vi "overheat.vi"(8 "input valid":bool=TRUE, 9 "ready for output (T)":bool=TRUE, 10 "x":fxp<+/-,32,16>) -> (0 "output valid":bool, 1 "ready for input":bool, 2 "Output":fxp<+/-,32,16>)   [LabVIEW 2018]
uses:
  <vilib>/rvi/FXPMathLib/FxpDiv/subVIs/nifxpmath_Div_SimConfig.ctl
  <vilib>/rvi/FXPMathLib/FxpDiv/simVIs/DllFxpDivTemp_sub.vi
  <vilib>/rvi/FXPMathLib/FxpDiv/XNode/nifxpmath_Div.xnode
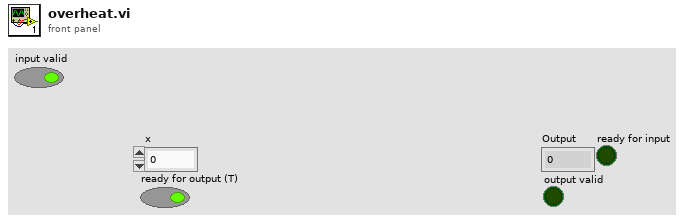
[diagram p1: front panel]
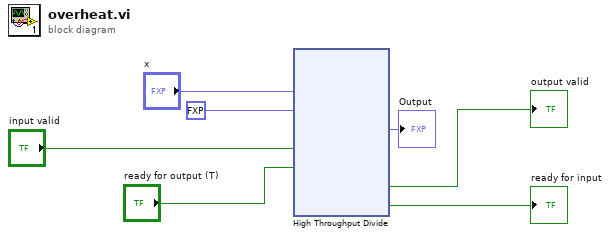
[diagram p0: block diagram]
diagram:
  n1 = xnode "High Throughput Divide"("x"="x", "y"=fxp<+,2,2> 2.0, "input valid"="input valid", "ready for output (T)"="ready for output (T)") -> ("x/y"=→"Output":fxp<+/-,32,16>, "output valid"=→"output valid":bool, "ready for input"=→"ready for input":bool)
